vi "ContourManual2001.vi"   [LabVIEW 2013]
uses:
  ModeType.ctl
  <vilib>/Heliosphere Research LLC/Advanced Plotting Toolkit/api_plotting/Contour_Manual.vi
  <vilib>/Heliosphere Research LLC/Advanced Plotting Toolkit/Advanced Plotting Toolkit.lvlib
types:
  T1 = typedef "ModeType.ctl" = enum16{"Normal", "Expected Failure", "Skipped", "Broken"}
  T2 = typedef "Advanced Plotting Toolkit.lvlib/PlotID.ctl" = i32
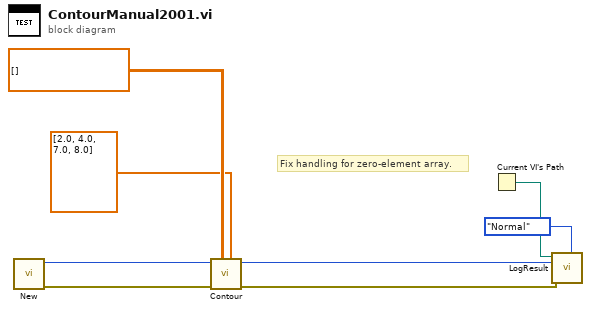
[diagram p0: block diagram]
diagram:
  # "Fix handling for zero-element array."
  n1 = call <vilib>:"New.vi"() -> ("error out"=w6:errorcluster, "Plot ID"=w7:T2)  [unwired: 10 in]
  n2 = call-poly <vilib>:"Contour.vi"("Levels"=dbl[] [2.0, 4.0, 7.0, 8.0], "Z Data"=dbl[][] [], "error in (no error)"=w6, "Plot ID"=w7) -> ("error out"=w4:errorcluster, "Plot ID Out"=w5:T2)  [unwired: 6 in]
  n3 = Current VI's Path() -> (path=w8:path)
  n4 = call "LogResult.vi"("Mode"=ModeType."Normal", "Test Result"=w4, "Test Artifact"=w5, "VI Path"=w8) -> ()  [unwired: 8 in]
